vi "2L07-lambda_de_periode_n0.vi"(0 "t":dbl[](array[numeric]), 1 "dN(t)":dbl[](array[numeric]), 2 "N(t)":dbl[](array[numeric]), 3 "t 1":dbl, 4 "t 2":dbl) -> (5 "dN(t1-t2)":dbl, 6 "N(t1)":dbl, 7 "La (t1-t2)":dbl)   [LabVIEW 2010, in "lv_02.lvlib"]
doc: "A partir de la série t, dN, N(t), le VI calcule sur une période t1-t2 \n- les survivants à t1\n- les effectifs défaillants dN(t1 à t2)\n- la durée de la période dt\n- le taux de défaillance qui en résulte"
uses:
  lv_02.lvlib
panel:
  out "dt":dbl
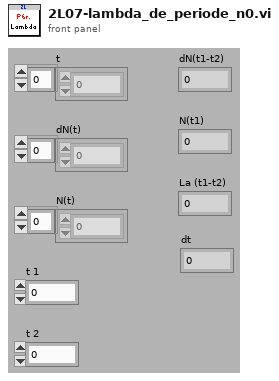
[diagram p1: front panel]
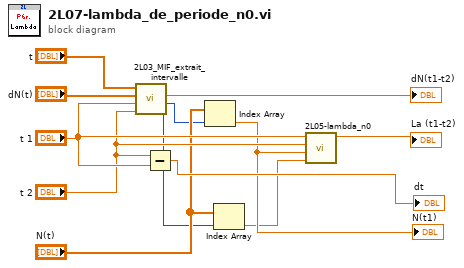
[diagram p0: block diagram]
diagram:
  n1 = call "2L03_MIF_extrait_intervalle.vi"("X fin"="t 2", "X deb"="t 1", "N"="dN(t)", "X"="t") -> ("i fin"=w1:i32, "i deb"=w4:i32, "Cumul"=→"dN(t1-t2)":dbl)  [unwired: 2 in, 3 out]
  n2 = Subtract(x="t 2", y="t 1") -> (x-y=→"dt":dbl)
  n3 = Index Array(array="N(t)", index=w4) -> (element=w3:dbl)
  "N(t1)" <- w3
  n4 = Index Array(array="N(t)", index=w1) -> (element=w2:dbl)
  n5 = call "2L05-lambda_n0.vi"("N(tfin)"=w2, "N(tdeb)"=w3, "tfin"="t 2", "tdeb"="t 1") -> ("lambda"=→"La (t1-t2)":dbl)  [unwired: 4 in, 1 out]
